vi "Finish Move.vi"(8 "error in (no error)":errorcluster, 11 "ScrollingList in":refnum<class "ScrollingList.lvclass">) -> (0 "error out":errorcluster, 3 "ScrollingList out":refnum<class "ScrollingList.lvclass">)   [LabVIEW 2020, in "ScrollingList.lvclass"]
uses:
  ScrollingList.lvclass
  C:/Program Files/National Instruments/LabVIEW 2020/vi.lib/QSI/QControls/QControl Classes/Picture/Picture.lvclass
  ScrollingList.lvclass/ScrollingList.ctl
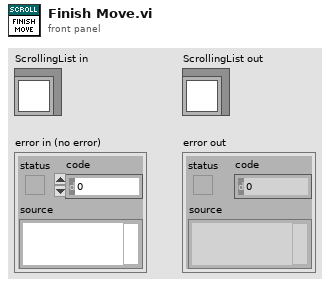
[diagram p1: front panel]
types:
  T1 = typedef "LVMouseTypeDef.ctl" = cluster{"Mouse Position":cluster{"X":i32, "Y":i32}, "Mouse Modifiers":cluster{"Button Down":bool, "Shift Mod":bool, "Menu Mod":bool, "Option Mod":bool}}
  T2 = typedef "ScrollingList.lvclass/State Data.ctl" = cluster{"Timeout":i32, "Time":timestamp, "Y":i32, "Origin:Top":i16, "Rate":dbl, "ListItems":string[], "Item Height":i32, "Max Height":i32}
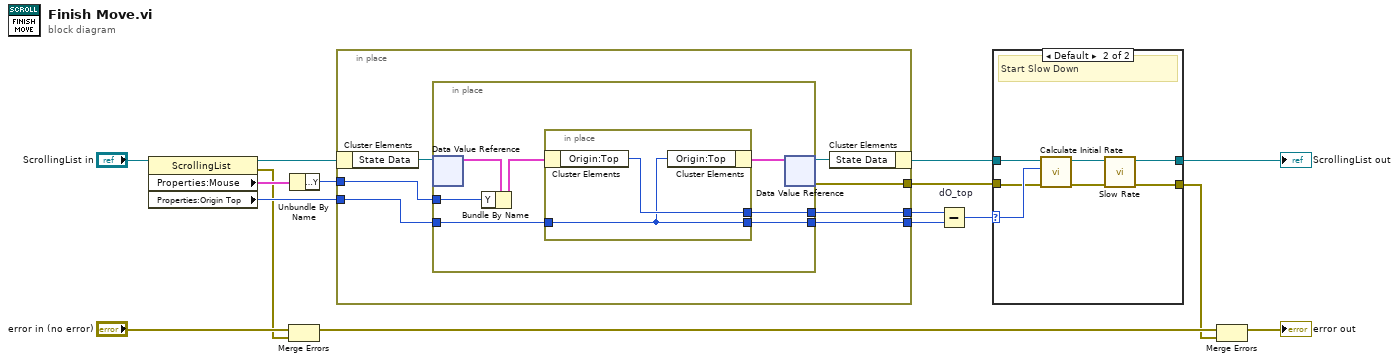
[diagram p0: block diagram]
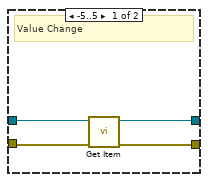
[diagram p2: hidden frame]
diagram:
  n1 = property on="Property Node" class="ScrollingList"(reference="ScrollingList in") -> (reference out=w13:refnum<class "ScrollingList.lvclass">, error out=w3:errorcluster, "Properties:Mouse"=w14:T1, "Properties:Origin Top"=w11:i16)  [unwired: 1 in]
  n2 = Merge Errors("error in (no error)", w3) -> (w4:errorcluster)
  n3 = Unbundle By Name(w14) -> ("Mouse Position.Y"=w12:i32)
  n4 = in-place {
    in-place-border: w12 -> [w22]
    in-place-border: w11 -> [w21]
    in-place-border: [w19] -> w10
    in-place-border: [w18] -> w9
    in-place-border: [w17] -> w5
    n5 = in-place-cluster #1(w13) -> ("State Data"=w23:refnum<data-value>)
    n6 = in-place {
      in-place-border: w22 -> [w24]
      in-place-border: w21 -> [w29]
      in-place-border: [w28] -> w19
      in-place-border: [w27] -> w18
      n7 = in-place-dvr #2(w23) -> (w26:T2)  [unwired: 1 out]
      n8 = Bundle By Name(cluster=w26, "Y"=w24) -> (w25:T2)
      n9 = in-place {
        in-place-border: [w32] -> w28
        in-place-border: w29 -> [w31]
        in-place-border: [w31] -> w27
        n10 = in-place-cluster #3(w25) -> ("Origin:Top"=w32:i16)
        n11 = in-place-cluster #3("Origin:Top"=w31) -> (w30:T2)
      }
      n12 = in-place-dvr #2(w30) -> (w20:refnum<data-value>, w17:errorcluster)
    }
    n13 = in-place-cluster #1("State Data"=w20) -> (w8:refnum<class "ScrollingList.lvclass">)
  }
  n14 = Subtract "dO_top"(x=w10, y=w9) -> (x-y=w6:i16)
  n15 = case shown="Default" w6 {
    selector: w6 -> [_ w42]
    tunnel: w8 -> [w36 w43]
    tunnel: [w35 w38] -> w7
    tunnel: w5 -> [w34 w41]
    tunnel: [w33 w37] -> w1
    frame -5..5 {
      # "Value Change"
      n16 = call "Get Item.vi"("error in (no error)"=w34, "ScrollingList in"=w36) -> ("error out"=w33:errorcluster, "ScrollingList (dup)"=w35:refnum<class "ScrollingList.lvclass">)  [unwired: 8 in]
    }
    frame Default {
      # "Start Slow Down"
      n17 = call "Calculate Initial Rate.vi"("error in (no error)"=w41, "Position Change"=w42, "ScrollingList in"=w43) -> ("error out"=w39:errorcluster, "ScrollingList (dup)"=w40:refnum<class "ScrollingList.lvclass">)  [unwired: 7 in]
      n18 = call "Slow Rate.vi"("error in (no error)"=w39, "ScrollingList in"=w40) -> ("error out"=w37:errorcluster, "ScrollingList out"=w38:refnum<class "ScrollingList.lvclass">)  [unwired: 8 in]
    }
  }
  "ScrollingList out" <- w7
  n19 = Merge Errors(w4, w1) -> (→"error out":errorcluster)
